vi "AO Configure Trigger.vi"(8 "error in (no error)":errorcluster, 10 "Params":variant, 11 "NI Analog Output in":refnum<class "NI Analog Output.lvclass">) -> (0 "error out":errorcluster, 3 "NI Analog Output out":refnum<class "NI Analog Output.lvclass">)   [LabVIEW 2020, in "NI DAQmx.lvlib" / "NI Analog Output.lvclass"]
uses:
  NI Analog Output.lvclass
  D:/WSGitHub/RTFWK/Realization/NI DAQmx Base/NI DAQmx Base.lvclass
  TypeDefs/Trigger Config.ctl
  <vilib>/DAQmx/configure/trigger.llb/DAQmx Start Trigger (None).vi
  <vilib>/DAQmx/configure/trigger.llb/DAQmx Start Trigger (Analog Edge).vi
  <vilib>/DAQmx/configure/trigger.llb/DAQmx Start Trigger (Digital Edge).vi
  <resource>/objmgr/daqmx.rc
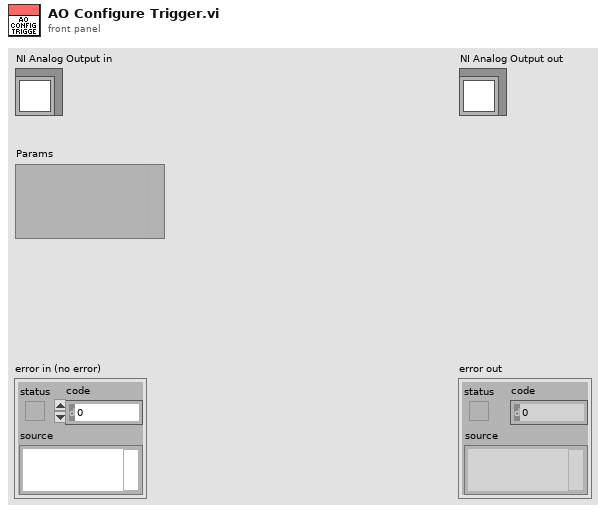
[diagram p1: front panel]
types:
  T1 = typedef "Trigger Config.ctl" = cluster{"trigger type":string, "source":string, "slope":i32, "analog level":dbl, "analog hysteresis":dbl}
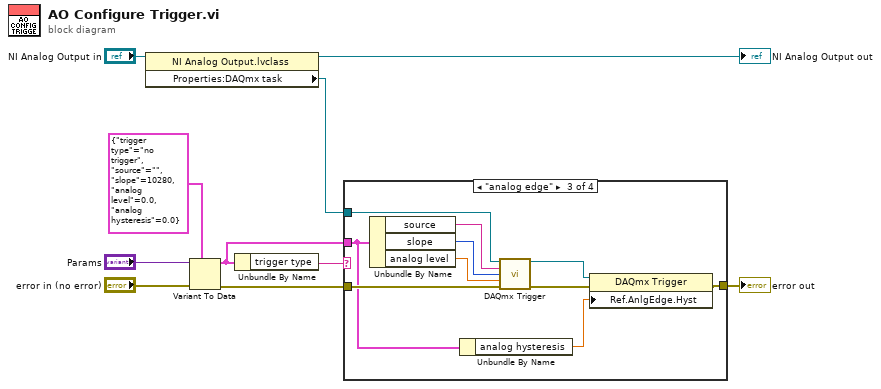
[diagram p0: block diagram]
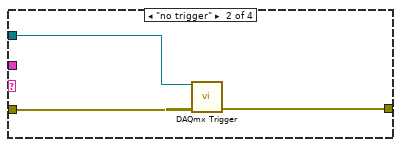
[diagram p3: hidden frame]
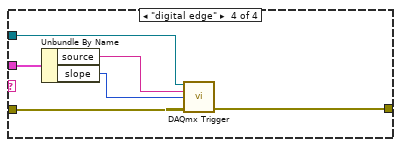
[diagram p4: hidden frame]
diagram:
  n1 = property class="NI Analog Output.lvclass"(reference="NI Analog Output in") -> (reference out=→"NI Analog Output out":refnum<class "NI Analog Output.lvclass">, "Properties:DAQmx task"=w7:refnum<k21>)  [unwired: 1 in, 1 out]
  n2 = Variant To Data(error in="error in (no error)", type=T1 {"trigger type"="no trigger", "source"="", "slope"=10280, "analog level"=0.0, "analog hysteresis"=0.0}, Variant="Params") -> (data=w1:T1, error out=w5:errorcluster)
  n3 = Unbundle By Name(w1) -> ("trigger type"=w2:string)
  n4 = case shown="\"analog edge\"" w2 {
    tunnel: [w11 w14 w17 w30] -> w9
    tunnel: w7 -> [_ w13 w23 w29]
    tunnel: w5 -> [w11 w12 w24 w28]
    tunnel: w1 -> [_ _ w16 w27]
    frame Default {
      # "invalid type"
    }
    frame "no trigger" {
      n5 = call-poly <vilib>:"DAQmx Trigger.vi"("task/channels in"=w13, "error in"=w12) -> ("error out"=w14:errorcluster)  [unwired: 12 in, 1 out]
    }
    frame "analog edge" {
      n6 = Unbundle By Name(w16) -> ("source"=w22:string, "slope"=w21:i32, "analog level"=w20:dbl)
      n7 = Unbundle By Name(w16) -> ("analog hysteresis"=w15:dbl)
      n8 = call-poly <vilib>:"DAQmx Trigger.vi"("task/channels in"=w23, "source"=w22, "slope"=w21, "level"=w20, "error in"=w24) -> ("task out"=w18:refnum<k21>, "error out"=w19:errorcluster)  [unwired: 9 in]
      n9 = property class="DAQmx Trigger"(reference=w18, error in=w19, "Ref.AnlgEdge.Hyst"=w15) -> (error out=w17:errorcluster)  [unwired: 1 out]
    }
    frame "digital edge" {
      n10 = Unbundle By Name(w27) -> ("source"=w25:string, "slope"=w26:i32)
      n11 = call-poly <vilib>:"DAQmx Trigger.vi"("task/channels in"=w29, "source"=w25, "edge"=w26, "error in"=w28) -> ("error out"=w30:errorcluster)  [unwired: 10 in, 1 out]
    }
  }
  "error out" <- w9
